vi "XYZ Test.vi"() -> ()   [LabVIEW 2014]
uses:
  XYZ Stage Control.ctl
  support/Instrument Status.ctl
  XYZ Coordinate Control.ctl
  XYZ Function.ctl
  XYZ Refnums.ctl
  XYZ Connection Settings.ctl
panel:
  in  "stop":bool
  in  "OK Button":bool
  in  "Function":T1
  out "Position":dbl[](array[numeric])
  in  "Coordinate Control":T2
  out "Instrument Status":T3
  in  "Manual Control":T4 {"Z step" scale=0.1..10.0; "XY Step" scale=0.1..1000.0}
  # "LICENSED MATERIALS – PROPERTY OF IBM\nCopyright IBM Corp. 2016,\nALL RIGHTS RESERVED"
  # "XY"
  # "Z"
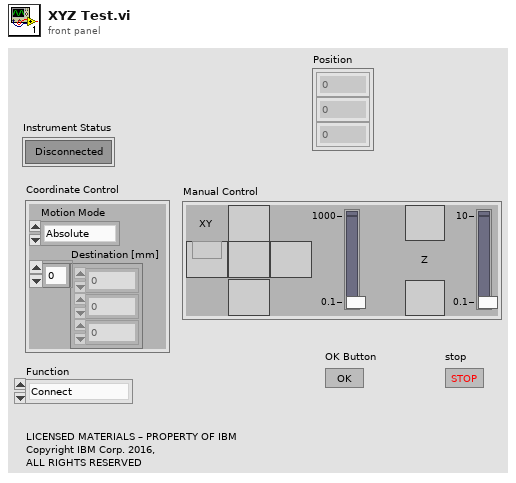
[diagram p1: front panel]
types:
  T1 = typedef "XYZ Function.ctl" = enum16{"Connect", "Initialize", "Calibrate", "Meaure Range", "Limits", "Center", "Set Zero", "Velocity", "Manual Control", "Coordinate Move", "Move with Backlash Compensation", "Meander", "Sequence", "Analog Output", "Send Command", "Show Protocol", "Get Status", "Disconnect", "Update Refnums"}
  T2 = typedef "XYZ Coordinate Control.ctl" = cluster{"Motion Mode":enum16{"Absolute", "Relative"}, "Destination [mm]":dbl[]}
  T3 = typedef "Instrument Status.ctl" = bool
  T4 = typedef "XYZ Stage Control.ctl" = cluster{"North":bool, "South":bool, "West":bool, "East":bool, "Up":bool, "Down":bool, "Stop":bool, "XY Step":dbl, "Z step":dbl}
  T5 = typedef "XYZ Connection Settings.ctl" = cluster{"Tango VISA":refnum<visa-resource-name>, "Baudrate":i32, "Show Protocol?":bool}
  T6 = typedef "XYZ Refnums.ctl" = cluster{"Instrument Status":refnum<vi>, "Position":refnum<vi>, "Manual Control":refnum<vi>, "Up":refnum<vi>, "Down":refnum<vi>, "North":refnum<vi>, "South":refnum<vi>, "East":refnum<vi>, "West":refnum<vi>, "Stop":refnum<vi>, "Limits":refnum<vi>}
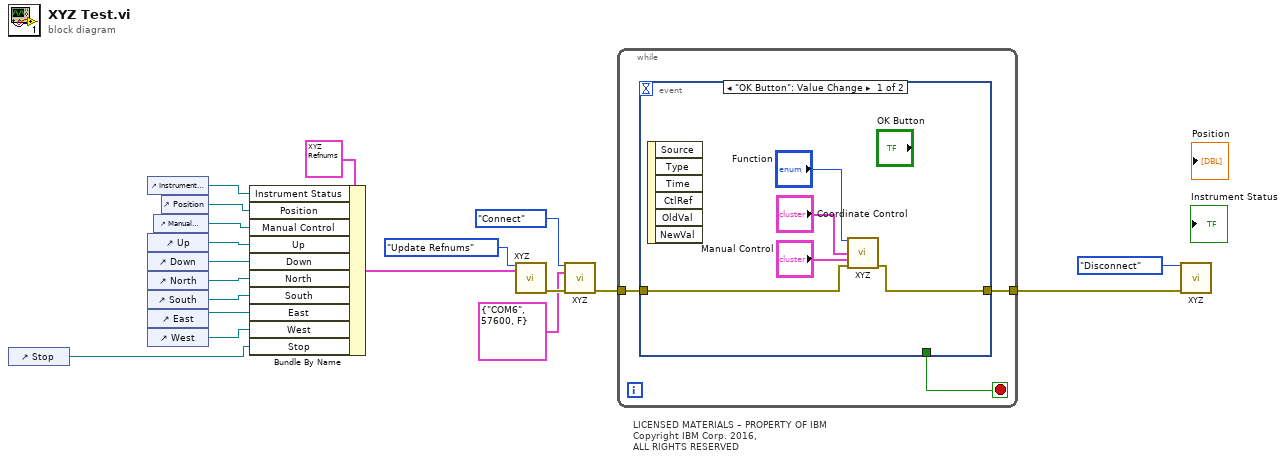
[diagram p0: block diagram]
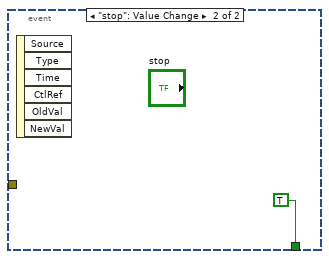
[diagram p2: hidden frame]
diagram:
  # "LICENSED MATERIALS – PROPERTY OF IBM\nCopyright IBM Corp. 2016,\nALL RIGHTS RESERVED"
  n1 = control-ref of="Stop"() -> (w1:refnum<vi>)
  n2 = control-ref of="Instrument Status"() -> (w17:refnum<vi>)
  n3 = control-ref of="Up"() -> (w14:refnum<vi>)
  n4 = control-ref of="Down"() -> (w13:refnum<vi>)
  n5 = control-ref of="North"() -> (w12:refnum<vi>)
  n6 = control-ref of="South"() -> (w11:refnum<vi>)
  n7 = control-ref of="East"() -> (w2:refnum<vi>)
  n8 = control-ref of="West"() -> (w10:refnum<vi>)
  n9 = control-ref of="Manual Control"() -> (w15:refnum<vi>)
  n10 = control-ref of="Position"() -> (w16:refnum<vi>)
  n11 = Bundle By Name(cluster=T6 {"Instrument Status"=refnum, "Position"=refnum, "Manual Control"=refnum, "Up"=refnum, "Down"=refnum, "North"=refnum, "South"=refnum, "East"=refnum, "West"=refnum, "Stop"=refnum, "Limits"=refnum} ("Refnums"), "Instrument Status"=w17, "Position"=w16, "Manual Control"=w15, "Up"=w14, "Down"=w13, "North"=w12, "South"=w11, "East"=w2, "West"=w10, "Stop"=w1) -> (w18:T6)
  n12 = call "XYZ.vi"("Function"=XYZ_Function."Update Refnums", "Refnums"=w18) -> ("Error Out"=w7:errorcluster)  [unwired: 11 in, 2 out]
  n13 = call "XYZ.vi"("Function"=XYZ_Function."Connect", "Connection Settings"=T5 {"Tango VISA"="COM6", "Baudrate"=57600, "Show Protocol?"=FALSE}, "Error In (no error)"=w7) -> ("Error Out"=w4:errorcluster)  [unwired: 10 in, 2 out]
  n14 = while {
    tunnel: w4 -> [w22]
    tunnel: [w21] -> w3
    stop <- w20 stop-if-true
    n15 = event shown="[0] \"OK Button\": Value Change" {
      selector: _ -> [_ _]
      dyn-events: _ -> [_ _]
      timeout: _ -> [_ _]
      tunnel: w22 -> [w24 _]
      tunnel: [w23 _] -> w21
      tunnel: [_ TRUE] -> w20
      event "OK Button": Value Change {
        n16 = event-data() -> ()  [unwired: 1 in, 6 out]
        n17 = call "XYZ.vi"("Function"="Function", "Coordinate Control"="Coordinate Control", "Manual Control"="Manual Control", "Error In (no error)"=w24) -> ("Error Out"=w23:errorcluster)  [unwired: 9 in, 2 out]
      }
      event "stop": Value Change {
        n18 = event-data() -> ()  [unwired: 1 in, 6 out]
      }
    }
  }
  n19 = call "XYZ.vi"("Function"=XYZ_Function."Disconnect", "Error In (no error)"=w3) -> ()  [unwired: 11 in, 3 out]
